vi "LinearSystemId_CreateDriveTrainVelocitySystem.vi"(4 "G":dbl, 6 "JKgMetersSquared":dbl, 8 "rbMeters":dbl, 9 "rMeters":dbl, 10 "MassKg":dbl, 11 "Motor":T1 {"Jr_KgM2" format="%13.5p"; "L_H" format="%13.5p"; "Kt_NMPerAmp" format="%13.5p"; "KvINV_RadPerSecPerVolt" format="%13.5p"; "R_Ohms" format="%13.5p"; "FreeSpeed_RadPerSec" format="%13.5p"; "FreeCurrent_Amps" format="%13.5p"; "StallCurrent_Amps" format="%13.5p"; "StallTorque_NM" format="%13.5p"; "nominalVoltage_Volts" format="%13.5p"}) -> (0 "Size Coerced":bool, 3 "Linearsystem":T2)   [LabVIEW 2019, in "Trajectory_Library.lvlib"]
doc: "Create a state-space model of a differential drive drivetrain. In this model, the states are [v_left, v_right]?, inputs are [V_left, V_right]? and outputs are [v_left, v_right]?.\n\nInputs: \n - motor -- the gearbox representing the motors driving the drivetrain.\n - massKg -- the mass of the robot.\n - rMeters -- the radius of the wheels in meters.\n - rbMeters -- the radius of the base (half the track width) in meters.\n - JKgMetersSquared -- the moment of inertia of the robot.\n - G -- the gearing reduction as output over input.\n\nOutputs:\n - LinearSystem -- A LinearSystem cluster representing a differential drivetrain.\n - SizeCoerced -- A boolean indicating that sizes had to be adjusted. A value of TRUE indicates an error."
uses:
  Trajectory_Library.lvlib
  LINEAR_SYSTEM.ctl
  <vilib>/Analysis/Matrix/Datatypes/RealMatrix.ctl
  DCMOTOR.CTL
  <vilib>/Analysis/Matrix/NI_Matrix.lvlib
panel:
  # "<States,States>"
  # "<States,Inputs>"
  # "<Outputs,States>"
  # "<Outputs,Inputs>"
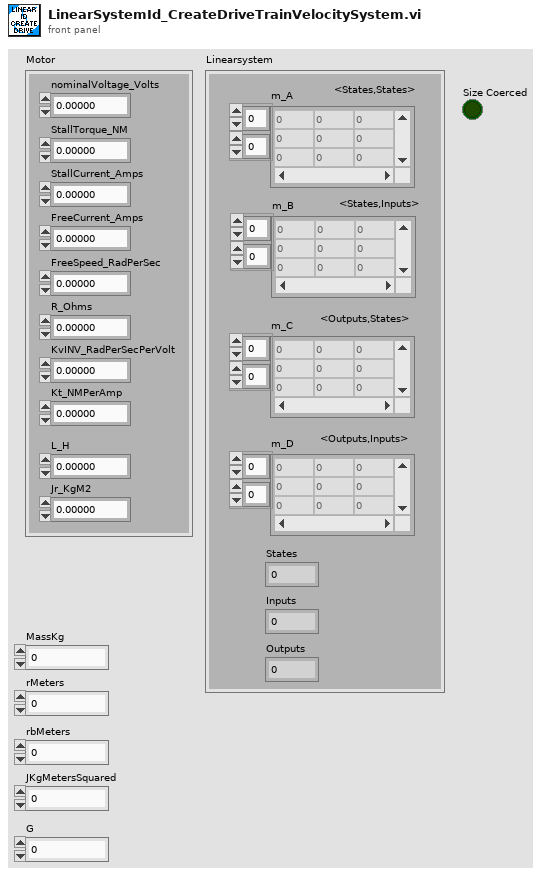
[diagram p1: front panel]
types:
  T1 = typedef "Trajectory_Library.lvlib/DCMOTOR.CTL" = cluster{"nominalVoltage_Volts":dbl, "StallTorque_NM":dbl, "StallCurrent_Amps":dbl, "FreeCurrent_Amps":dbl, "FreeSpeed_RadPerSec":dbl, "R_Ohms":dbl, "KvINV_RadPerSecPerVolt":dbl, "Kt_NMPerAmp":dbl, "L_H":dbl, "Jr_KgM2":dbl}
  T2 = typedef "Trajectory_Library.lvlib/LINEAR_SYSTEM.ctl" = cluster{"m_A":T3, "m_B":T3, "m_C":T3, "m_D":T3, "States":i32, "Inputs":i32, "Outputs":i32}
  T3 = typedef "NI_Matrix.lvlib/RealMatrix.ctl" = dbl[][]
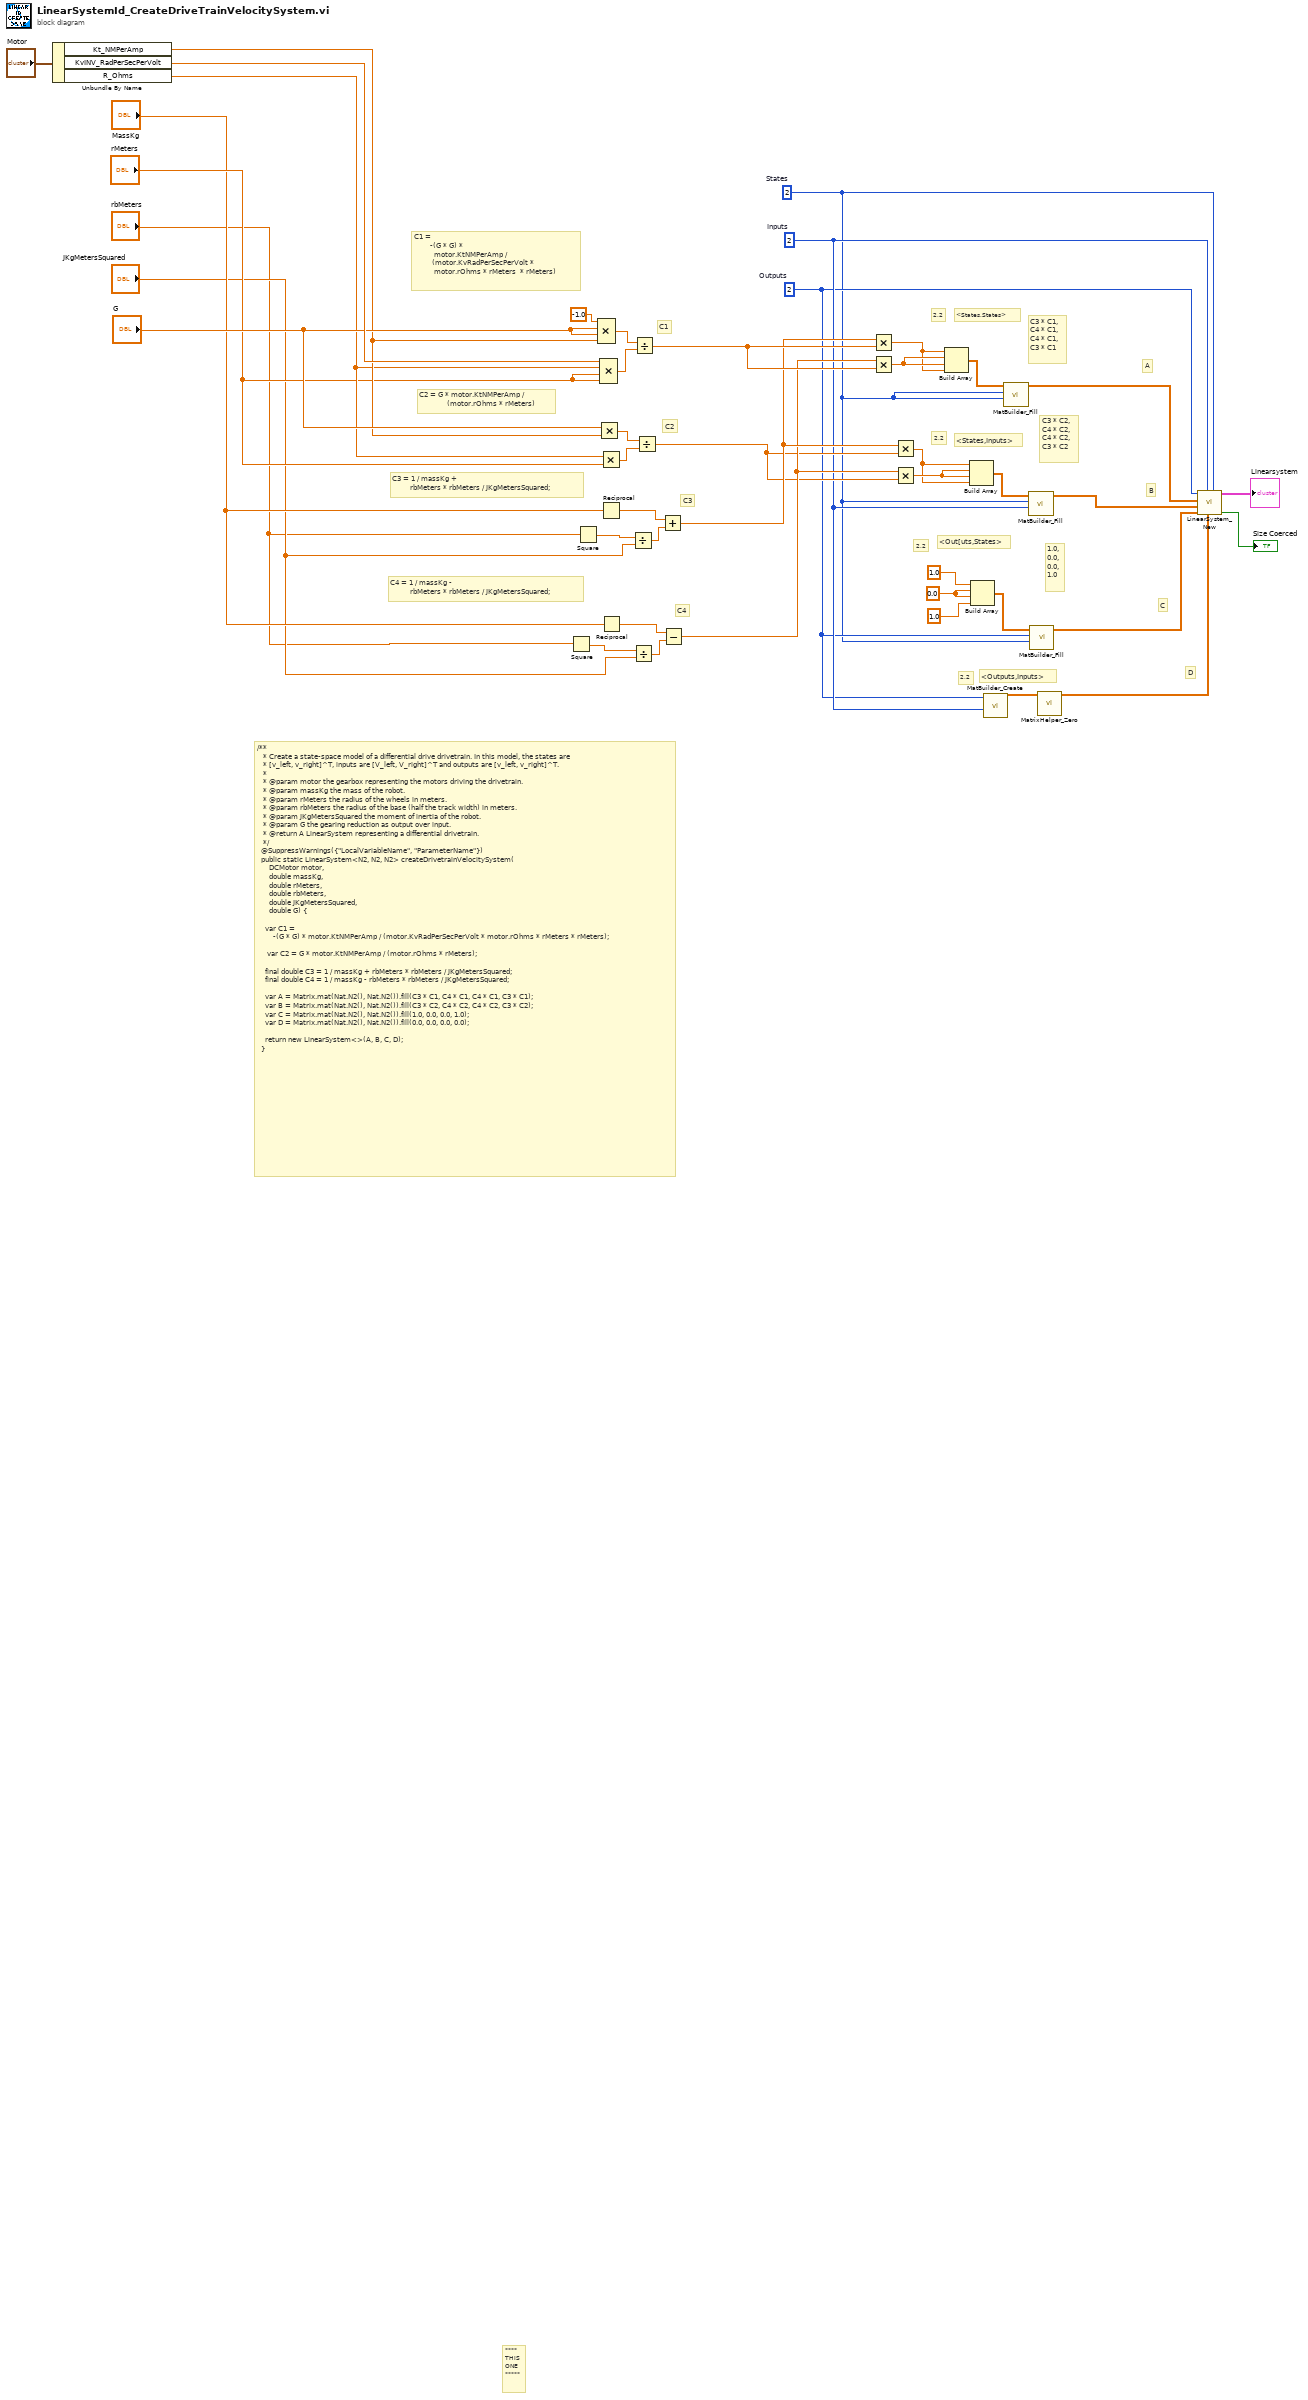
[diagram p0: block diagram]
diagram:
  w8 = 2  # Outputs
  w17 = 2  # Inputs
  w7 = 2  # States
  w11 = 0.0 ("element")
  # "1.0, \n0.0, \n0.0, \n1.0"
  # "C3 * C2, \nC4 * C2, \nC4 * C2, \nC3 * C2"
  # "C3 * C1, \nC4 * C1, \nC4 * C1, \nC3 * C1"
  # "D"
  # "C"
  # "B"
  # "A"
  # "C4 = 1 / massKg - \n          rbMeters * rbMeters / JKgMetersSquared;"
  # "C3 = 1 / massKg + \n         rbMeters * rbMeters / JKgMetersSquared;"
  # "C2 = G * motor.KtNMPerAmp / \n              (motor.rOhms * rMeters)"
  # "C1 =\n        -(G * G) *\n          motor.KtNMPerAmp / \n         (motor.KvRadPerSecPerVolt * \n          motor.rOhms * rMeters  * rMeters)"
  # "C4"
  # "C3"
  # "C2"
  # "C1"
  # "2,2"
  # "2,2"
  # "2,2"
  # "2,2"
  # "<States,States>"
  # "<States,Inputs>"
  # "<Out[uts,States>"
  # "<Outputs,Inputs>"
  # "/**\n   * Create a state-space model of a differential drive drivetrain. In this model, the states are\n   * [v_left, v_right]^T, inputs are [V_left, V_right]^T and outputs are [v_left, v_right]^T.\n   *\n   * @param motor the gearbox representing the motors driving the drivetrain.\n   * @param massKg the mass of the robot.\n   * @param rMeters the radius of the wheels in meters.\n   * @param rbMeters the radius of the base (half the track width) in meters.\n   * @param JKgMetersSquared the moment of inertia of the robot.\n   * @param G the gearing reduction as output over input.\n   * @return A LinearSystem representing a differential drivetrain.\n   */\n  @SuppressWarnings({\"LocalVariableName\", \"ParameterName\"})\n  public static LinearSystem<N2, N2, N2> createDrivetrainVelocitySystem(\n      DCMotor motor,\n      double massKg,\n      double rMeters,\n      double rbMeters,\n      double JKgMetersSquared,\n      double G) {\n\n    var C1 =\n        -(G * G) * motor.KtNMPerAmp / (motor.KvRadPerSecPerVolt * motor.rOhms * rMeters * rMeters);\n    \n     var C2 = G * motor.KtNMPerAmp / (motor.rOhms * rMeters);\n\n    final double C3 = 1 / massKg + rbMeters * rbMeters / JKgMetersSquared;\n    final double C4 = 1 / massKg - rbMeters * rbMeters / JKgMetersSquared;\n\n    var A = Matrix.mat(Nat.N2(), Nat.N2()).fill(C3 * C1, C4 * C1, C4 * C1, C3 * C1);\n    var B = Matrix.mat(Nat.N2(), Nat.N2()).fill(C3 * C2, C4 * C2, C4 * C2, C3 * C2);\n    var C = Matrix.mat(Nat.N2(), Nat.N2()).fill(1.0, 0.0, 0.0, 1.0);\n    var D = Matrix.mat(Nat.N2(), Nat.N2()).fill(0.0, 0.0, 0.0, 0.0);\n\n    return new LinearSystem<>(A, B, C, D);\n  }"
  # "****\nTHIS\nONE\n*****"
  n1 = Unbundle By Name("Motor") -> ("Kt_NMPerAmp"=w37:dbl, "KvINV_RadPerSecPerVolt"=w41:dbl, "R_Ohms"=w34:dbl)
  n2 = Square(x="rbMeters") -> (x^2=w1:dbl)
  n3 = Square(x="rbMeters") -> (x^2=w3:dbl)
  n4 = Compound Arithmetic op=MULTIPLY(-1.0 ("value"), "G", "G", w37) -> (w40:dbl)
  n5 = Multiply(x="G", y=w37) -> (x*y=w36:dbl)
  n6 = Multiply(x=w34, y="rMeters") -> (x*y=w35:dbl)
  n7 = Reciprocal(x="MassKg") -> (1/x=w32:dbl)
  n8 = Compound Arithmetic op=MULTIPLY(w41, w34, "rMeters", "rMeters") -> (w39:dbl)
  n9 = Reciprocal(x="MassKg") -> (1/x=w30:dbl)
  n10 = Divide(x=w3, y="JKgMetersSquared") -> (x/y=w31:dbl)
  n11 = Divide(x=w1, y="JKgMetersSquared") -> (x/y=w29:dbl)
  n12 = Divide(x=w40, y=w39) -> (x/y=w26:dbl)
  n13 = Divide(x=w36, y=w35) -> (x/y=w23:dbl)
  n14 = Add(x=w32, y=w31) -> (x+y=w25:dbl)
  n15 = Subtract(x=w30, y=w29) -> (x-y=w24:dbl)
  n16 = Multiply(x=w25, y=w26) -> (x*y=w21:dbl)
  n17 = Multiply(x=w24, y=w26) -> (x*y=w22:dbl)
  n18 = Multiply(x=w25, y=w23) -> (x*y=w15:dbl)
  n19 = Multiply(x=w24, y=w23) -> (x*y=w16:dbl)
  n20 = Build Array(w21, w22, w22, w21) -> (w20:dbl[])
  n21 = Build Array(w15, w16, w16, w15) -> (w18:dbl[])
  n22 = Build Array(1.0 ("element"), w11, w11, 1.0 ("element")) -> (w13:dbl[])
  n23 = call "MatBuilder_Create.vi"("Columns"=w17, "Rows"=w8) -> ("output matrix"=w6:T3)  [unwired: 9 in]
  n24 = call "MatBuilder_Fill.vi"("Columns"=w7, "Rows"=w7, "Value List"=w20) -> ("output matrix"=w19:T3)  [unwired: 8 in]
  n25 = call "MatBuilder_Fill.vi"("Columns"=w17, "Rows"=w7, "Value List"=w18) -> ("output matrix"=w14:T3)  [unwired: 8 in]
  n26 = call "MatBuilder_Fill.vi"("Columns"=w7, "Rows"=w8, "Value List"=w13) -> ("output matrix"=w9:T3)  [unwired: 8 in]
  n27 = call "MatrixHelper_Zero.vi"("input matrix"=w6) -> ("output matrix"=w5:T3)  [unwired: 10 in]
  n28 = call "LinearSystem_New.vi"("States"=w7, "D"=w5, "Inputs"=w17, "C"=w9, "B"=w14, "A"=w19, "Outputs"=w8) -> ("Size Coerced"=→"Size Coerced":bool, "Linearsystem"=→"Linearsystem":T2)  [unwired: 3 in]
